vi "WLAN - TV - RW - UTIL - PowerLevel(dBm_milli-dBm).vi"(0 "Power Level(dBm)":dbl) -> (4 "Coherced Power(milli-dBm)":i32, 6 "Coherced Power(dBm)":dbl)   [LabVIEW 2011]
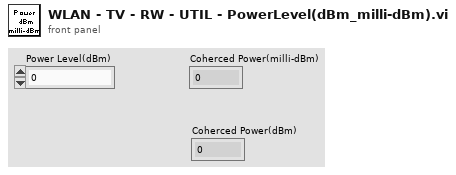
[diagram p1: front panel]
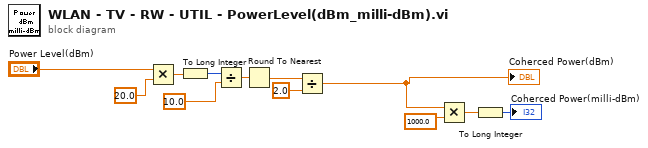
[diagram p0: block diagram]
diagram:
  n1 = Multiply(x="Power Level(dBm)", y=20.0) -> (x*y=w12:dbl)
  n2 = To Long Integer(number=w12) -> (32bit integer=w11:i32)
  n3 = Divide(x=w11, y=10.0) -> (x/y=w8:dbl)
  n4 = Round To Nearest(number=w8) -> (nearest integer value=w3:dbl)
  n5 = Divide(x=w3, y=2.0) -> (x/y=w1:dbl)
  "Coherced Power(dBm)" <- w1
  n6 = Multiply(x=w1, y=1000.0) -> (x*y=w6:dbl)
  n7 = To Long Integer(number=w6) -> (32bit integer=→"Coherced Power(milli-dBm)":i32)
